vi "GetCursorsPositionsFromTemperatureGraph.vi"(8 "error in (no error)":errorcluster, 11 "Temperature Profile 2":refnum<vi>) -> (0 "error out":errorcluster, 1 "End Index":dbl, 2 "Start Index":dbl, 3 "Temperature Profile 3":refnum<vi>)   [LabVIEW 2015]
doc: "Use this template to build a VI to use as a subVI."
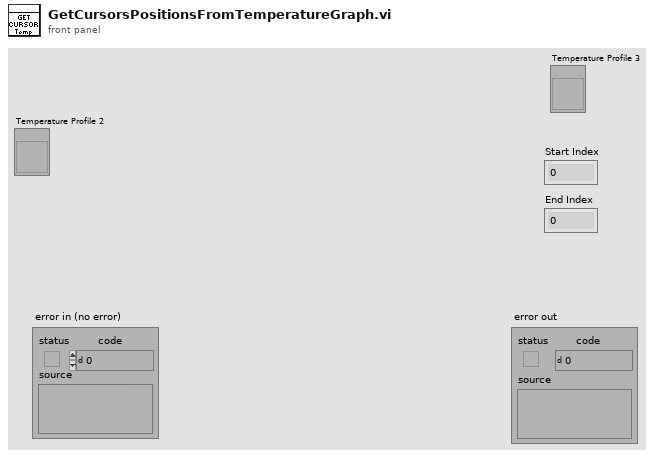
[diagram p1: front panel]
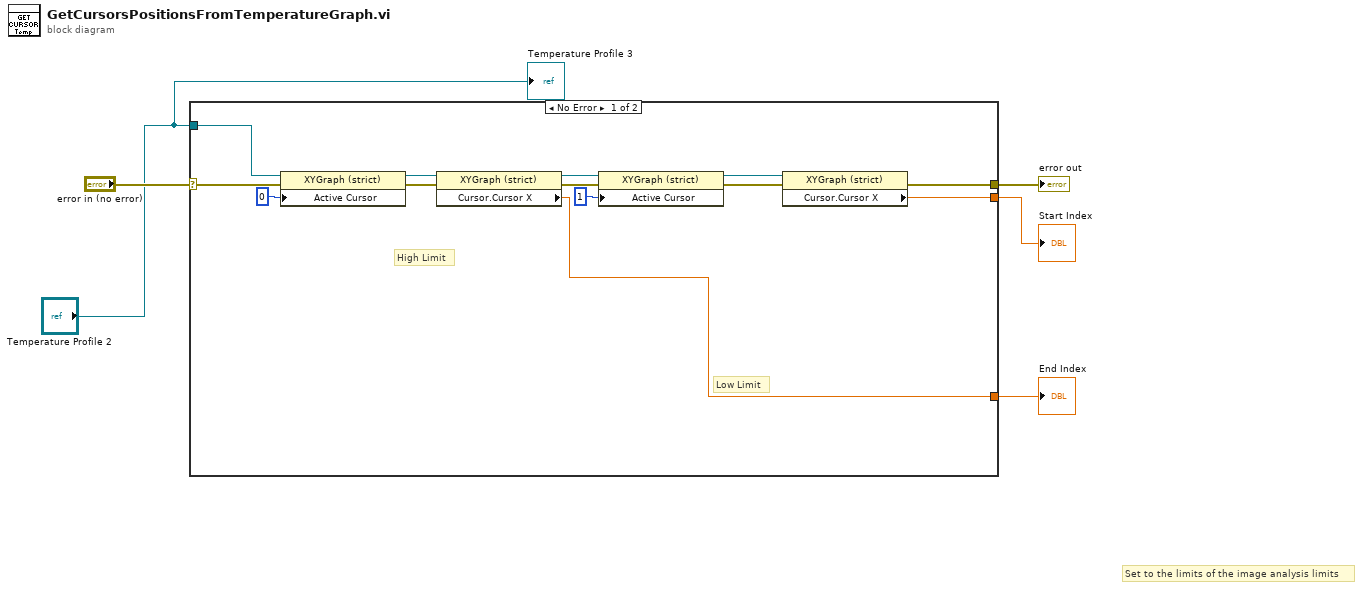
[diagram p0: block diagram]
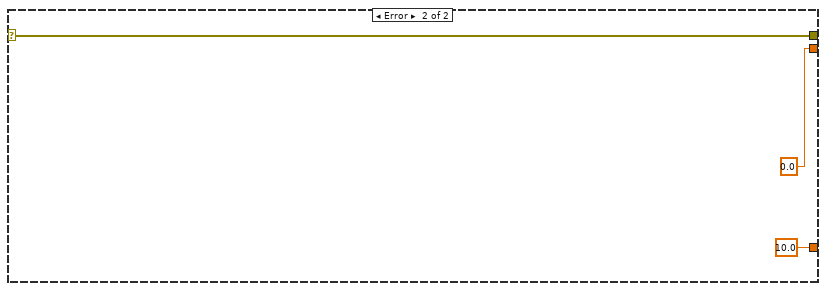
[diagram p2: hidden frame]
diagram:
  # "Set to the limits of the image analysis limits"
  n1 = case shown="No Error" "error in (no error)" {
    selector: "error in (no error)" -> [w9 w21]
    tunnel: [w10 w21] -> w4
    tunnel: "Temperature Profile 2" -> [w11 _]
    tunnel: [w7 10.0 ("Cursor.Cursor X")] -> w3
    tunnel: [w8 0.0 ("Cursor.Cursor X")] -> w2
    frame No Error {
      # "Low Limit"
      # "High Limit"
      n2 = property class="XYGraph (strict)"(reference=w11, error in=w9, "Active Cursor"=u32 0) -> (reference out=w6:refnum<vi>, error out=w15:errorcluster)
      n3 = property class="XYGraph (strict)"(reference=w6, error in=w15) -> (reference out=w16:refnum<vi>, error out=w14:errorcluster, "Cursor.Cursor X"=w7:dbl)
      n4 = property class="XYGraph (strict)"(reference=w16, error in=w14, "Active Cursor"=u32 1) -> (reference out=w13:refnum<vi>, error out=w12:errorcluster)
      n5 = property class="XYGraph (strict)"(reference=w13, error in=w12) -> (error out=w10:errorcluster, "Cursor.Cursor X"=w8:dbl)  [unwired: 1 out]
    }
    frame Error {
    }
  }
  "error out" <- w4
  "Start Index" <- w2
  "End Index" <- w3
  "Temperature Profile 3" <- "Temperature Profile 2"
